vi "Configure Signal Path.vi"(8 "error in (no error)":errorcluster, 9 "Instance (1)":i32=1, 10 "Signal Path (Port1.IFIn)":i32(ring)=1 items=["Port1.IFIn"=1, "Port2.IFIn"=2, "Port3.IFIn"=3], 11 "VISA resource name":refnum<visa-resource-name>) -> (0 "error out":errorcluster, 3 "VISA resource name out":refnum<visa-resource-name>)   [LabVIEW 2020, in "Rohde&Schwarz CMP LR WPAN Measurement.lvlib"]
doc: "Selects the signal path for the measured RF signal.\nValid Values:\nPort1.IFln, Port2.IFln, Port3.IFln\n\nAttribute:\nRSCMPLRWM_ATTR_SIGNAL_PATH\n\nRemote-control command:\nROUTe:WPAN:MEAS<i>:SPATh"
uses:
  <instrlib>/Rohde&Schwarz CMP LR WPAN Measurement/Rohde&Schwarz CMP LR WPAN Measurement.lvlib
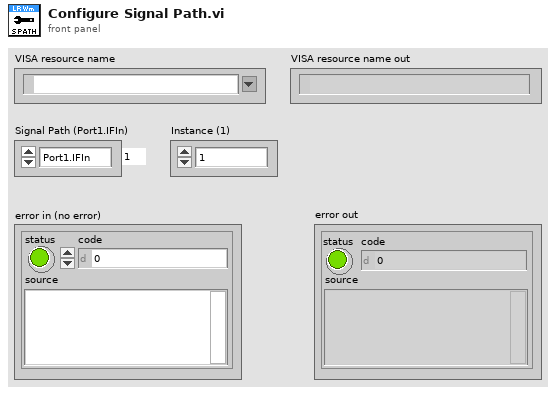
[diagram p1: front panel]
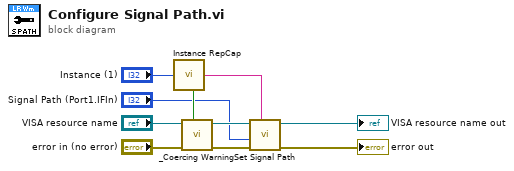
[diagram p0: block diagram]
diagram:
  n1 = call <instrlib>:"Instance RepCap.vi"("Instance In"="Instance (1)") -> ("In Range?"=w7:bool, "RepCap Identifier Out"=w8:string)  [unwired: 1 in]
  n2 = call <instrlib>:"_Coercing Warning.vi"("In Range?"=w7, "error in (no error)"="error in (no error)", "VISA resource name"="VISA resource name") -> ("error out"=w4:errorcluster, "VISA resource name out"=w3:refnum<visa-resource-name>)  [unwired: 7 in]
  n3 = call "Set Signal Path"("Repeated Capabilities"=w8, "error in (no error)"=w4, "Signal Path (1 - Port1.IFIn)"="Signal Path (Port1.IFIn)", "instrument handle"=w3) -> ("error out"=→"error out":errorcluster, "instrument handle out"=→"VISA resource name out":refnum<visa-resource-name>)  [unwired: 6 in]
